vi "Next Terminal Task.vi"(8 "error in (no error)":errorcluster, 10 "Composite Task In":refnum<class "Task Ancestor.lvclass">, 11 "Iterator in":refnum<class "Composite Task Iterator.lvclass">) -> (0 "error out":errorcluster, 1 "Next Task Out":refnum<class "Task Ancestor.lvclass">, 2 "Composite Task Out":refnum<class "Task Ancestor.lvclass">, 3 "Iterator out":refnum<class "Composite Task Iterator.lvclass">, 4 "Last":bool)   [LabVIEW 2024, in "Composite Task Iterator.lvclass"]
uses:
  Composite Task Iterator.lvclass
  Ancestor Class/Task/Task Ancestor/Task Ancestor.lvclass
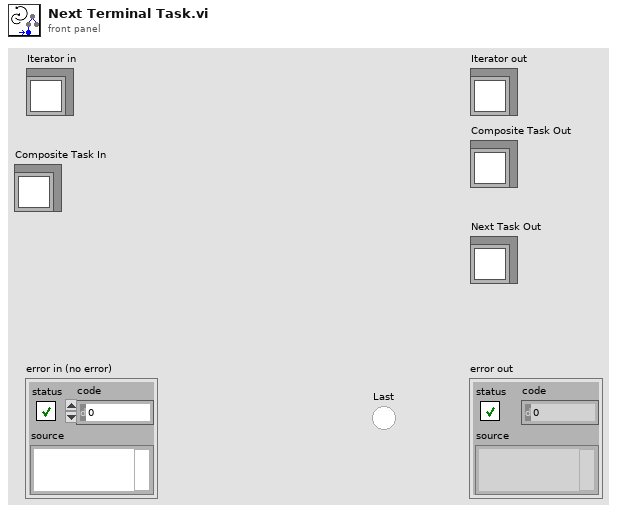
[diagram p1: front panel]
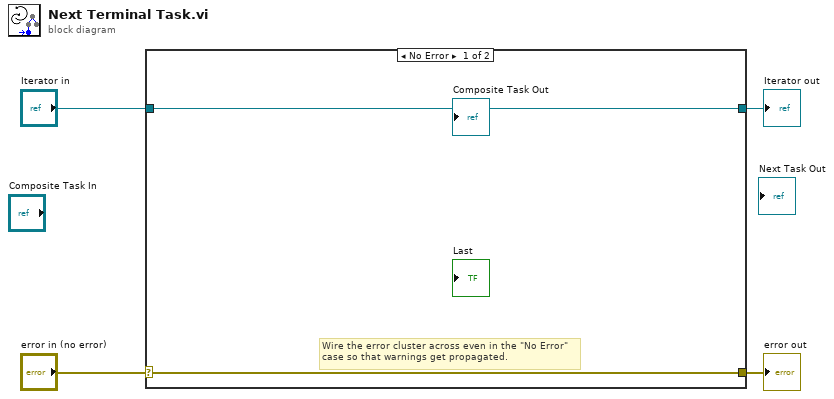
[diagram p0: block diagram]
diagram:
  n1 = case shown="No Error" "error in (no error)" {
    selector: "error in (no error)" -> [w5 w8]
    tunnel: [w5 w8] -> w3
    tunnel: [w6 w7] -> w1
    tunnel: "Iterator in" -> [w6 w7]
    frame No Error {
      # "Wire the error cluster across even in the \"No Error\"\ncase so that warnings get propagated."
    }
    frame Error {
    }
  }
  "error out" <- w3
  "Iterator out" <- w1
